vi "HumanExecute.vi"(8 "error in (no error)":errorcluster) -> (0 "error out":errorcluster)   [LabVIEW 2023]
doc: "Execute for Human\n\ninput:\n error in (cluster)\n\noutput:\n error out (cluster)"
uses:
  <vilib>/Rock Robotics/WPI/Joystick/XBox Axes Indexer.ctl
  <vilib>/Rock Robotics/WPI/Joystick/XBox Buttons Indexer.ctl
  <vilib>/Rock Robotics/WPI/ThirdParty/JAS_Junk/TrajLib/MathUtil_ApplyDeadband.vi
  <vilib>/Rock Robotics/WPI/ThirdParty/JAS_Junk/TrajLib/VI/DigSeqLogic_Edge_On.vi
  <vilib>/Rock Robotics/WPI/ThirdParty/JAS_Junk/TrajLib/VI/BoolCmd_Send_Internal.vi
  <vilib>/Rock Robotics/WPI/ThirdParty/JAS_Junk/TrajLib/VI/BoolCmd_ObtainQueue.vi
  HumanGlobal.vi
  <vilib>/Rock Robotics/Network Tables/NT Write String.vi
  <vilib>/Rock Robotics/WPI/ThirdParty/JAS_Junk/TrajLib/Trajectory_Library.lvlib
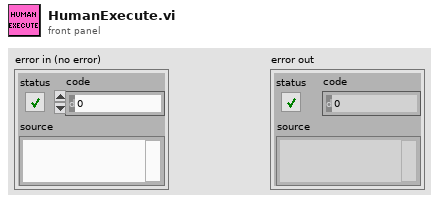
[diagram p1: front panel]
types:
  T1 = typedef "XBox Axes Indexer.ctl" = enum16{"Left X", "Left Y", "Left Trigger", "Right Trigger", "Right X", "Right Y"}
  T2 = typedef "XBox Buttons Indexer.ctl" = enum16{"A", "B", "X", "Y", "Left Bumper", "Right Bumper", "Back", "Start", "Left Joystick", "Right Joystick"}
  T3 = typedef "WPI_JoystickDevRef.ctl" = cluster{"Device":T4}
  T4 = typedef "WPI_JoystickDeviceEnum.ctl" = enum16{"USB 0", "USB 1", "USB 2", "USB 3", "USB 4", "USB 5"}
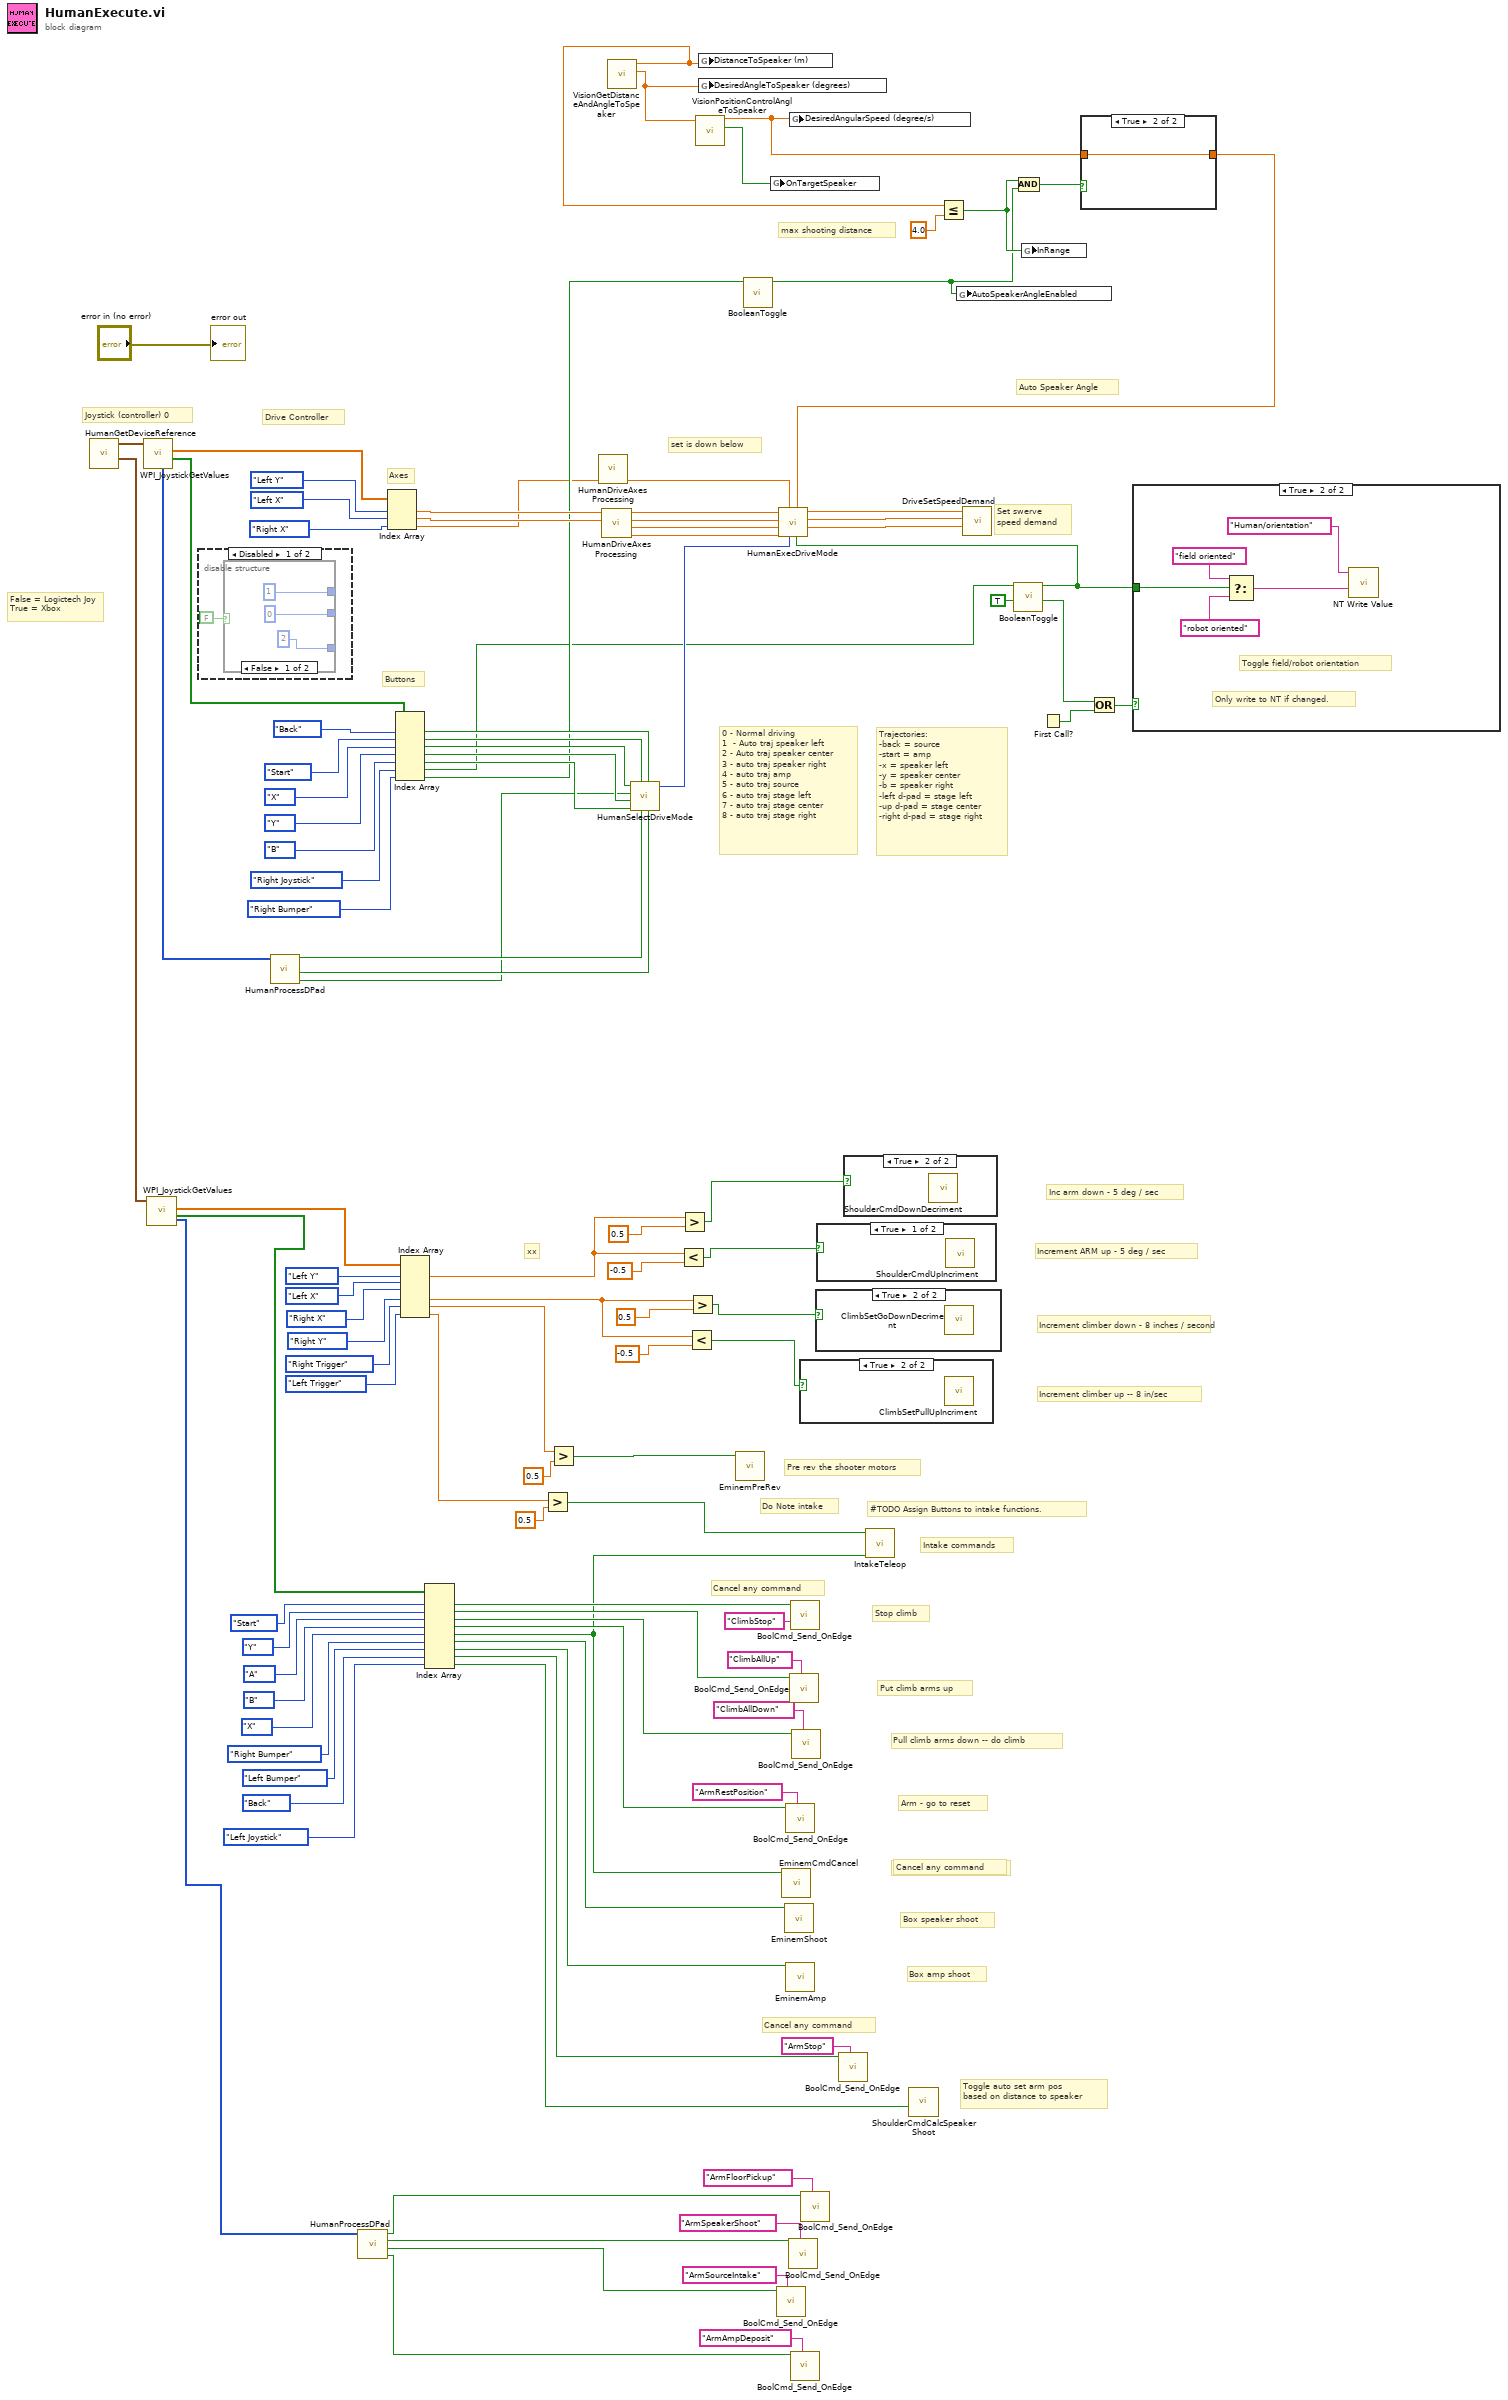
[diagram p0: block diagram]
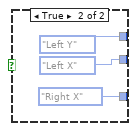
[diagram p3: hidden frame]
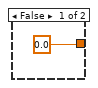
[diagram p5: hidden frame]
diagram:
  # "Intake commands"
  # "#TODO Assign Buttons to intake functions."
  # "Auto Speaker Angle"
  # "0 - Normal driving\n1  - Auto traj speaker left \n2 - Auto traj speaker center\n3 - auto traj speaker right \n4 - auto traj amp\n5 - auto traj source\n6 - auto traj stage left\n7 - auto traj stage center\n8 - auto traj stage right"
  # "False = Logictech Joy\nTrue = Xbox"
  # "Toggle auto set arm pos\nbased on distance to speaker"
  # "Box amp shoot"
  # "Box speaker shoot"
  # "Box - cancel any action"
  # "Arm - go to reset"
  # "Pull climb arms down -- do climb"
  # "Put climb arms up"
  # "Stop climb"
  # "Increment ARM up - 5 deg / sec"
  # "Increment climber up -- 8 in/sec"
  # "Do Note intake"
  # "Pre rev the shooter motors"
  # "max shooting distance"
  # "Increment climber down - 8 inches / second"
  # "xx"
  # "Cancel any command"
  # "Cancel any command"
  # "Inc arm down - 5 deg / sec"
  # "Trajectories:\n-back = source\n-start = amp\n-x = speaker left\n-y = speaker center\n-b = speaker right\n-left d-pad = stage left\n-up d-pad = stage center\n-right d-pad = stage right"
  # "Buttons"
  # "Axes"
  # "Cancel any command"
  # "set is down below"
  # "Set swerve\nspeed demand"
  # "Joystick (controller) 0"
  # "Drive Controller"
  n1 = call "HumanGetDeviceReference.vi"() -> ("Aux Joy"=w94:T3, "Driver Joy"=w98:T3)  [unwired: 9 in, 1 out]
  n2 = call <vilib>:"WPI_JoystickGetValues.vi"("JoystickDevRef"=w98) -> ("Buttons"=w73:bool[], "Axes"=w80:dbl[], "POVs"=w107:i16[])  [unwired: 6 in, 2 out]
  n3 = call <vilib>:"WPI_JoystickGetValues.vi"("JoystickDevRef"=w94) -> ("Buttons"=w84:bool[], "Axes"=w93:dbl[], "POVs"=w48:i16[])  [unwired: 6 in, 2 out]
  n4 = disable-structure shown="Disabled" {
    frame Disabled {
      n5 = case shown="False" FALSE {
        tunnel: [1 XBox_Axes_Indexer."Left Y" ("XBox Axes")] -> _
        tunnel: [0 XBox_Axes_Indexer."Left X" ("XBox Axes")] -> _
        tunnel: [2 XBox_Axes_Indexer."Right X" ("XBox Axes")] -> _
        frame False {
        }
        frame True {
        }
      }
    }
    frame Enabled {
    }
  }
  n6 = call "HumanProcessDPad.vi"("POV"=w107) -> ("Right"=w35:bool, "Left"=w36:bool, "Up"=w37:bool)  [unwired: 7 in, 1 out]
  n7 = call "HumanProcessDPad.vi"("POV"=w48) -> ("Right"=w45:bool, "Left"=w43:bool, "Down"=w44:bool, "Up"=w46:bool)  [unwired: 7 in]
  n8 = Index Array(array=w80, index #1=XBox_Axes_Indexer."Left Y" ("XBox Axes"), index #2=XBox_Axes_Indexer."Left X" ("XBox Axes"), index #3=XBox_Axes_Indexer."Right X" ("XBox Axes")) -> (element #1=w106:dbl, element #2=w105:dbl, element #3=w13:dbl)
  n9 = Index Array(array=w73, index #1=XBox_Buttons_Indexer."Back" ("Nothing"), index #2=XBox_Buttons_Indexer."Start" ("Nothing"), index #3=XBox_Buttons_Indexer."X" ("Nothing"), index #4=XBox_Buttons_Indexer."Y" ("Nothing"), index #5=XBox_Buttons_Indexer."B" ("Nothing"), index #6=XBox_Buttons_Indexer."Right Joystick" ("Nothing"), index #7=XBox_Buttons_Indexer."Right Bumper" ("Nothing")) -> (element #1=w42:bool, element #2=w41:bool, element #3=w40:bool, element #4=w39:bool, element #5=w38:bool, element #6=w6:bool, element #7=w20:bool)
  n10 = Index Array(array=w93, index #1=XBox_Axes_Indexer."Left Y" ("XBox Axes"), index #2=XBox_Axes_Indexer."Left X" ("XBox Axes"), index #3=XBox_Axes_Indexer."Right X" ("XBox Axes"), index #4=XBox_Axes_Indexer."Right Y" ("XBox Axes"), index #5=XBox_Axes_Indexer."Right Trigger" ("XBox Axes"), index #6=XBox_Axes_Indexer."Left Trigger" ("XBox Axes")) -> (element #1=w62:dbl, element #4=w54:dbl, element #5=w78:dbl, element #6=w75:dbl)  [unwired: 2 out]
  n11 = Index Array "Index Array"(array=w84, index #1=XBox_Buttons_Indexer."Start" ("Nothing"), index #2=XBox_Buttons_Indexer."Y" ("OpenCloseClaw"), index #3=XBox_Buttons_Indexer."A" ("GrabberIn"), index #4=XBox_Buttons_Indexer."B" ("GrabberOut"), index #5=XBox_Buttons_Indexer."X" ("Nothing"), index #6=XBox_Buttons_Indexer."Right Bumper" ("Nothing"), index #7=XBox_Buttons_Indexer."Left Bumper" ("Nothing"), index #8=XBox_Buttons_Indexer."Back" ("Place Cone"), index #9=XBox_Buttons_Indexer."Left Joystick" ("Place Cone")) -> (element #1=w53:bool, element #2=w52:bool, element #3=w51:bool, element #4=w50:bool, element #5=w1:bool, element #6=w79:bool, element #7=w74:bool, element #8=w49:bool, element #9=w14:bool)
  n12 = Greater?(x=w75, y=0.5) -> (0:w2:bool)
  n13 = Greater?(x=w78, y=0.5) -> (0:w17:bool)
  n14 = call "HumanDriveAxesProcessing.vi"("Right X"=w13) -> ("Right X"=w16:dbl)  [unwired: 7 in, 3 out]
  n15 = call "HumanDriveAxesProcessing.vi"("Left X"=w105, "Left Y"=w106) -> ("Right X"=w12:dbl, "Right Y"=w103:dbl, "Left X"=w104:dbl, "Left Y"=w102:dbl)  [unwired: 6 in]
  n16 = call "VisionGetDistanceAndAngleToSpeaker.vi"() -> ("DesiredAngle"=w28:dbl, "Distance"=w26:dbl)  [unwired: 10 in]
  n17 = call "HumanSelectDriveMode.vi"("AutoTrajStageLeft"=w36, "AutoTrajSource"=w42, "AutoTrajStageCenter"=w37, "AutoTrajAmp"=w41, "AutoTrajSpeakerRight"=w38, "AutoTrajSpeakerCenter"=w39, "AutoTrajStageRight"=w35, "AutoTrajSpeakerLeft"=w40) -> ("Drive Mode"=w34:i32)  [unwired: 3 in]
  n18 = Less?(x=w62, y=-0.5) -> (x < y?=w31:bool)
  n19 = Greater?(x=w62, y=0.5) -> (0:w30:bool)
  n20 = Less?(x=w54, y=-0.5) -> (x < y?=w33:bool)
  n21 = Greater?(x=w54, y=0.5) -> (0:w32:bool)
  n22 = call "VisionPositionControlAngleToSpeaker.vi"("TargetAngle"=w28) -> ("OnTargetSpeaker"=w27:bool, "DesiredAngularSpeed (degree/s)"=w24:dbl)  [unwired: 9 in]
  n23 = global write "HumanGlobal.vi" "DistanceToSpeaker (m)"(w26) -> ()
  n24 = global write "HumanGlobal.vi" "DesiredAngleToSpeaker (degrees)"(w28) -> ()
  n25 = call "EminemPreRev.vi"("PreRev"=w17) -> ()  [unwired: 10 in, 1 out]
  n26 = call "BooleanToggle.vi"("Toggle Edge In"=w20) -> ("Output"=w19:bool)  [unwired: 9 in, 1 out]
  n27 = global write "HumanGlobal.vi" "OnTargetSpeaker"(w27) -> ()
  n28 = call <vilib>:"BoolCmd_Send_OnEdge.vi"("Command Name"="ArmSourceIntake", "Value"=w43) -> ()  [unwired: 9 in, 1 out]
  n29 = call "EminemCmdCancel.vi"("box cancel"=w1) -> ()  [unwired: 11 in]
  n30 = call "EminemShoot.vi"("Box shoot"=w79) -> ()  [unwired: 10 in, 1 out]
  n31 = call <vilib>:"BoolCmd_Send_OnEdge.vi"("Command Name"="ArmRestPosition", "Value"=w50) -> ()  [unwired: 9 in, 1 out]
  n32 = call "EminemAmp.vi"("box amp"=w74) -> ()  [unwired: 11 in]
  n33 = call <vilib>:"BoolCmd_Send_OnEdge.vi"("Command Name"="ArmSpeakerShoot", "Value"=w44) -> ()  [unwired: 9 in, 1 out]
  n34 = global write "HumanGlobal.vi" "DesiredAngularSpeed (degree/s)"(w24) -> ()
  n35 = call <vilib>:"BoolCmd_Send_OnEdge.vi"("Command Name"="ClimbAllUp", "Value"=w52) -> ()  [unwired: 9 in, 1 out]
  n36 = call <vilib>:"BoolCmd_Send_OnEdge.vi"("Command Name"="ClimbStop", "Value"=w53) -> ()  [unwired: 9 in, 1 out]
  n37 = call <vilib>:"BoolCmd_Send_OnEdge.vi"("Command Name"="ArmAmpDeposit", "Value"=w45) -> ()  [unwired: 9 in, 1 out]
  n38 = call <vilib>:"BoolCmd_Send_OnEdge.vi"("Command Name"="ClimbAllDown", "Value"=w51) -> ()  [unwired: 9 in, 1 out]
  n39 = case shown="True" w33 {
    frame False {
    }
    frame True {
      n40 = call "ClimbSetPullUpIncriment.vi"() -> ()  [unwired: 11 in, 1 out]
    }
  }
  n41 = call <vilib>:"BoolCmd_Send_OnEdge.vi"("Command Name"="ArmFloorPickup", "Value"=w46) -> ()  [unwired: 9 in, 1 out]
  n42 = case shown="True" w32 {
    frame False {
    }
    frame True {
      n43 = call "ClimbSetGoDownDecriment.vi"() -> ()  [unwired: 11 in, 1 out]
    }
  }
  n44 = case shown="True" w31 {
    frame True {
      n45 = call "ShoulderCmdUpIncriment.vi"() -> ()  [unwired: 11 in, 1 out]
    }
    frame False {
    }
  }
  n46 = call <vilib>:"BoolCmd_Send_OnEdge.vi"("Command Name"="ArmStop", "Value"=w49) -> ()  [unwired: 9 in, 1 out]
  n47 = case shown="True" w30 {
    frame False {
    }
    frame True {
      n48 = call "ShoulderCmdDownDecriment.vi"() -> ()  [unwired: 11 in, 1 out]
    }
  }
  n49 = call "IntakeTeleop.vi"("CmdCancel"=w1, "CmdIntake"=w2) -> ()  [unwired: 10 in]
  n50 = call "ShoulderCmdCalcSpeakerShoot.vi"("ShoulderCmdCalcSpeaker"=w14) -> ()  [unwired: 10 in, 1 out]
  n51 = Less Or Equal?(x=w26, y=4.0) -> (x <= y?=w23:bool)
  n52 = global write "HumanGlobal.vi" "AutoSpeakerAngleEnabled"(w19) -> ()
  n53 = call "BooleanToggle.vi"("InitialState"=TRUE, "Toggle Edge In"=w6) -> ("Changed"=w3:bool, "Output"=w5:bool)  [unwired: 8 in]
  n54 = And(x=w23, y=w19) -> (x .and. y?=w22:bool)
  n55 = global write "HumanGlobal.vi" "InRange"(w23) -> ()
  n56 = First Call?() -> (First Call?: T/F=w7:bool)
  n57 = case shown="True" w22 {
    tunnel: w24 -> [_ w117]
    tunnel: [0.0 w117] -> w18
    frame False {
    }
    frame True {
    }
  }
  n58 = call "HumanExecDriveMode.vi"("Enable Field Oriented Drive"=w5, "AutoSpeakerAngle"=w18, "State"=w34, "Rotation"=w16, "Right X"=w12, "Right Y"=w103, "Left X"=w104, "Left Y"=w102) -> ("AMotorDemand"=w101:dbl, "YMotorDemand"=w100:dbl, "XMotorDemand"=w99:dbl)  [unwired: 1 in]
  n59 = call "DriveSetSpeedDemand.vi"("ASpeedDemand (d/s)"=w101, "YSpeedDemand (ft/s)"=w100, "XSpeedDemand (ft/s)"=w99) -> ()  [unwired: 9 in]
  n60 = Or(x=w3, y=w7) -> (x .or. y?=w8:bool)
  n61 = case shown="True" w8 {
    tunnel: w5 -> [_ w122]
    frame False {
    }
    frame True {
      # "Only write to NT if changed."
      # "Toggle field/robot orientation"
      n62 = Select(t="field oriented", s=w122, f="robot oriented") -> (s? t:f=w119:string)
      n63 = call-poly <vilib>:"NT Write Value.vi"("value"=w119, "name"="Human/orientation") -> ()  [unwired: 9 in, 1 out]
    }
  }
  "error out" <- "error in (no error)"
